vi "close.vi"(8 "error in (no error)":errorcluster, 11 "Instrument in":refnum<class "SR 830 & NI USB7855R.lvclass">) -> (0 "error out":errorcluster)   [LabVIEW 2020, in "SR 830 & NI USB7855R.lvclass"]
uses:
  SR 830 & NI USB7855R.lvclass
  SR 830 & NI USB7855R.lvclass/SR 830 & NI USB7855R.ctl
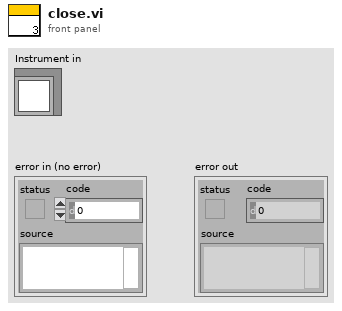
[diagram p1: front panel]
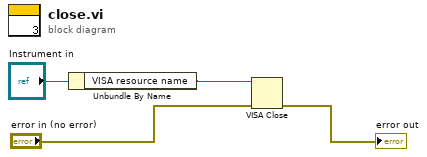
[diagram p0: block diagram]
diagram:
  n1 = Unbundle By Name("Instrument in") -> ("VISA resource name"=w3:refnum<visa-resource-name>)
  n2 = VISA Close(VISA resource name=w3, error in (no error)="error in (no error)") -> (error out=→"error out":errorcluster)
